vi "Intan_StreamData_64ch_parallelLoop.vi"(0 "VISA resource name":refnum<visa-resource-name>, 1 "refnum in":refnum<file>, 3 "stop":bool, 4 "Save Binary Data":bool, 5 "error in":errorcluster, 7 "byte order":T5(ring)=enum."little-endian", 8 "hdr fpath":path, 11 "DT_scale (sec)":dbl=0.01, 12 "aux file ref num":refnum<file>, 14 "save aux file":bool) -> (6 "N data scans to read (VISA)":i32=20, 10 "Nbytes VISA read":u32, 13 "VISA read iter":i32, 19 "error out":errorcluster)   [LabVIEW 2015]
doc: "Stream data to disk and user friendly display. Data is scaled and filtered prior to display.\n\nThis VI uses parallel while loop architecture: 1 loop reads from serial stream and saves raw bytes to disk; the other loop processes the data in chunk, scaling and filtering, then displays."
uses:
  zip_swcircularbuffer1_0_19b/Circular Buffer/Controls/Circular Buffer Status.ctl
  zip_swcircularbuffer1_0_19b/Circular Buffer/Controls/Circular Buffer Operations.ctl
  <vilib>/Utility/error.llb/DialogType.ctl
  zip_swcircularbuffer1_0_19b/Circular Buffer/Instance VIs/Circular Buffer(1D U16).vi
  zip_swcircularbuffer1_0_19b/Circular Buffer/Circular Buffer.lvlib
panel:
  out "A+B chans":i32[](array[numeric])
  out "Bchans":i32[](array[numeric])
  out "Achans":i32[](array[numeric])
  in  "Tab Control":T1(tab)
  in  "DisplayScale (uV/div)":u16(ring)=1 items=["6400", "3200", "1600", "800", "400", "200", "100", "50", "25"]
  in  "offset factor":dbl=1.0
  in  "Filter settings":T2={"LP Filter On/Off"=TRUE, "LP Cutoff (Hz)"=40.0, "HP Filter On/Off"=TRUE, "HP Cutoff (Hz)"=0.5, "Bandstop On/Off"=TRUE, "fl Cutoff (Hz)"=48.0, "fh Cutoff (Hz) "=52.0}
  out "Save status":bool
  out "non integer read":bool
  out "display iter":i32
  out "% buffer full":dbl(slide) scale=0.0..100.0
  in  "Ring Buffer Size":T3={"Samples per Channel"=640000, "Channels"=0}
  out "buffer underflow":bool
  out "Buffer Status  (read)":T4
  out "buffer overflow":bool
  out "Buffer Status (write)":T4
  in  "Center Traces":bool
  in  "Display Chans":i32[](listbox)=[1, 4, 13, 14, 15, 16, 17, 22]
  out "FS (Hz)":dbl
  in  "ChartDisplayLength (s)":dbl=5.0
  in  "Display Update interval (ms)":dbl=100.0
  in  "Buffer Read Interval (ms)":dbl=100.0
  in  "View Channels":u16(ring) items=["A and B (0-63)", "A chans (0-31)", "B chans (32-63)", "Free Select"]
  in  "bytes per scan":i32=140
  in  "Nchans":i32=64
  in  "start stream (Teensy char)":string="s"
  in  "pause stream (Teensy char)":string="p"
  out "Text response":string
  out "timestamp_array":i32[](array[numeric])
  out "aux_cmd_array":i32[][](array[numeric])
  out "binary data (from VISA read)":u16[](array[numeric])
  out "setscaleresult":dbl
  out "UpdateCode":i16
  out "xmax_init":dbl
  out "offset_init":dbl
  out "increment_init":dbl
  out "xmin_init":dbl
  out "NchansChanged":bool
  out "DispLengthChanged":bool
  out "XscaleRollover":bool
  out "error code out":i32 format="%0.0f"
  out "StopLoopsMaster":bool
  out "N_u16s  write to buf":i32
  out "Nelements to read from buf":dbl
  out "N data scans to display":u16=20
  out "YtxtLabelsAll":string[](array[string])
  out "Picture":picture
  out "Intan Streaming Data":dbl[][](graph)
  # "Intan-Teensy Bioelectric Module: Data Stream and Visualization"
  # "Display Settings"
  # "Ring Buffer Status"
  # "1-D data stream \nreformatted  to 2-D"
  # "xscale controls"
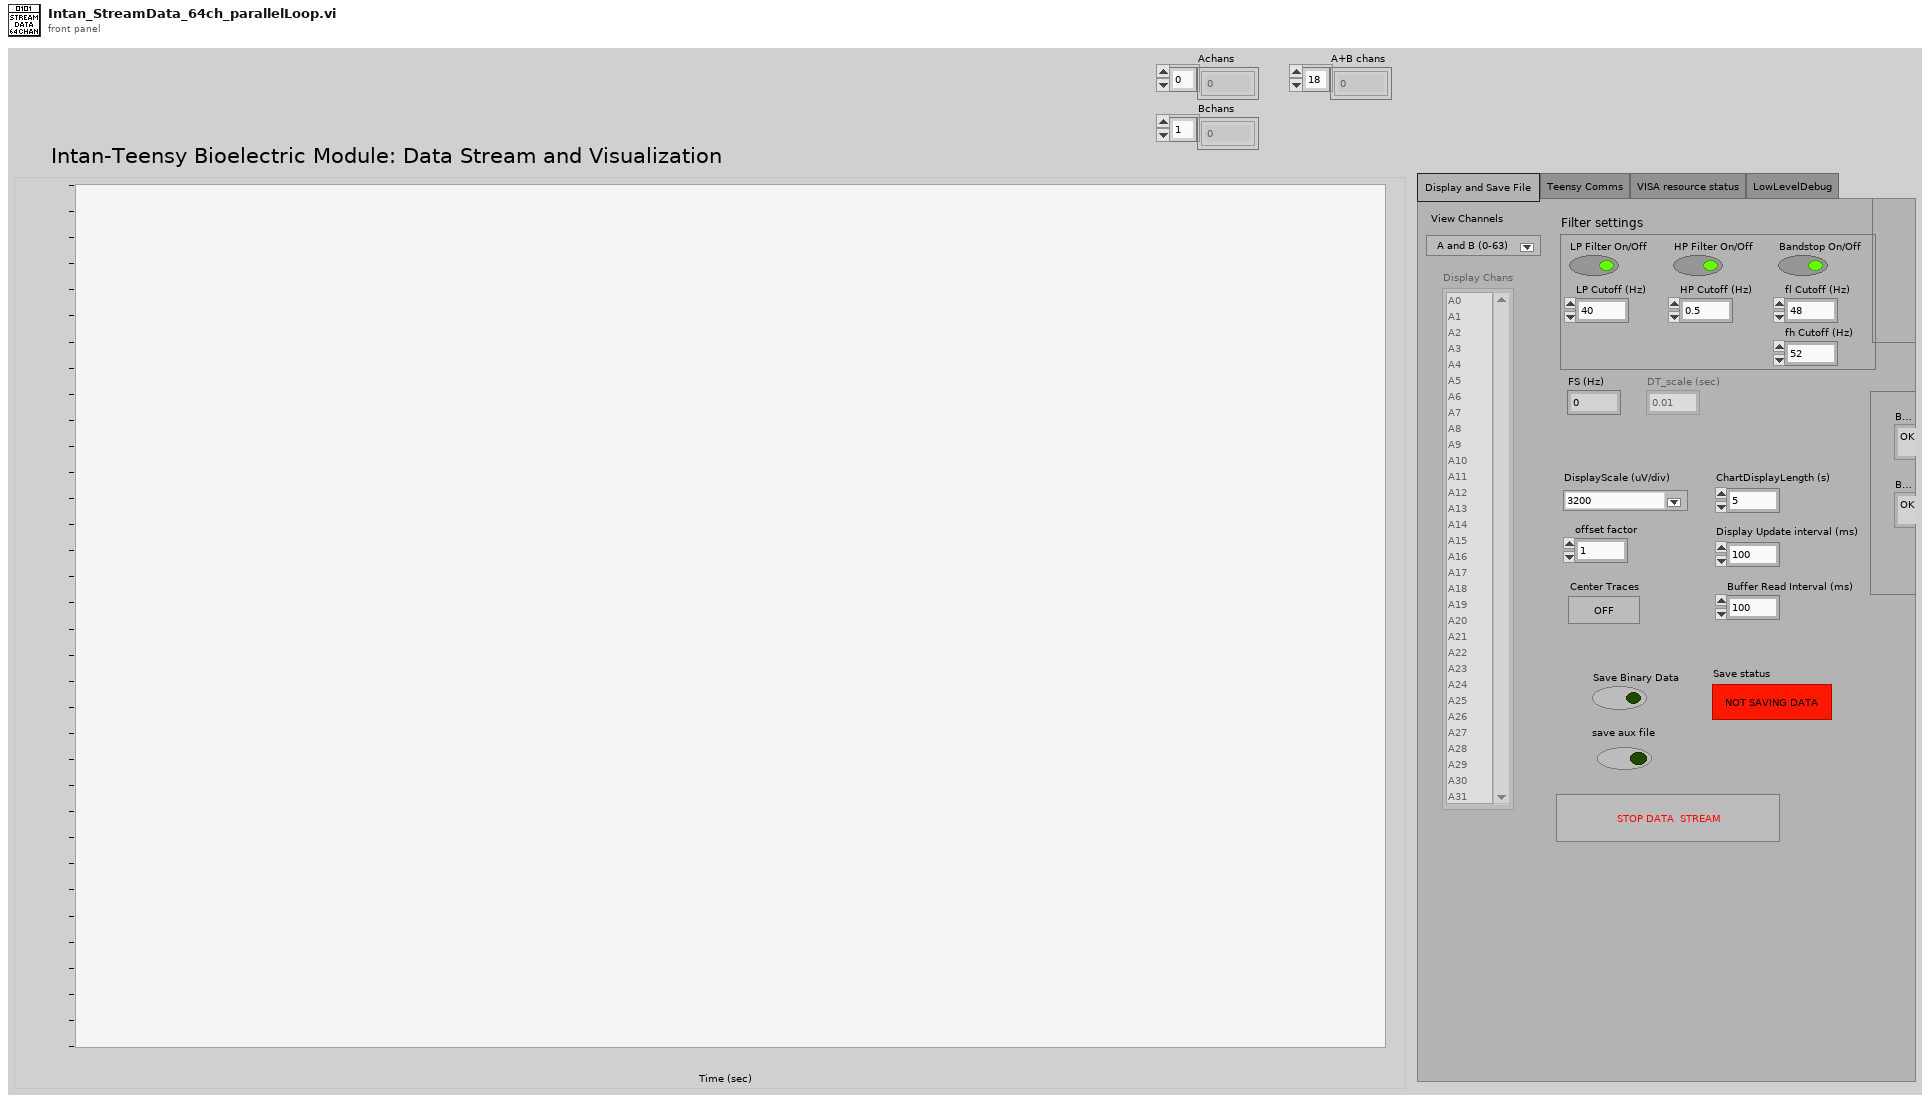
[diagram p1: front panel]
types:
  T1 = enum32{"Display and Save File ", "Teensy Comms", "VISA resource status", "LowLevelDebug"}
  T2 = cluster{"LP Filter On/Off":bool, "LP Cutoff (Hz)":dbl, "HP Filter On/Off":bool, "HP Cutoff (Hz)":dbl, "Bandstop On/Off":bool, "fl Cutoff (Hz)":dbl, "fh Cutoff (Hz) ":dbl}
  T3 = cluster{"Samples per Channel":u32, "Channels":u32}
  T4 = typedef "Circular Buffer.lvlib/Circular Buffer Status.ctl" = enum16{"OK", "Overflow", "Underflow"}
  T5 = enum16{"big-endian, network order", "native, host order", "little-endian"}
  T6 = typedef "Circular Buffer.lvlib/Circular Buffer Operations.ctl" = enum16{"Initialize", "Get Backlog", "Write", "Read (continuous)", "Read (most recent)"}
  T7 = enum8{"Enabled", "Disabled", "Disabled and Grayed Out"}
  T8 = typedef "LVRectTypeDef.ctl" = cluster{"Left":i16, "Top":i16, "Right":i16, "Bottom":i16}
  T9 = cluster{"XScale.Minimum":dbl, "XScale.Maximum":dbl, "XScale.Increment":dbl, "Nchannels":i32}
  T10 = cluster{"Maximum":dbl, dbl, dbl, dbl, dbl, dbl, "YscleMark":dbl, "Increment":dbl}
  T11 = typedef "DialogType.ctl" = u16
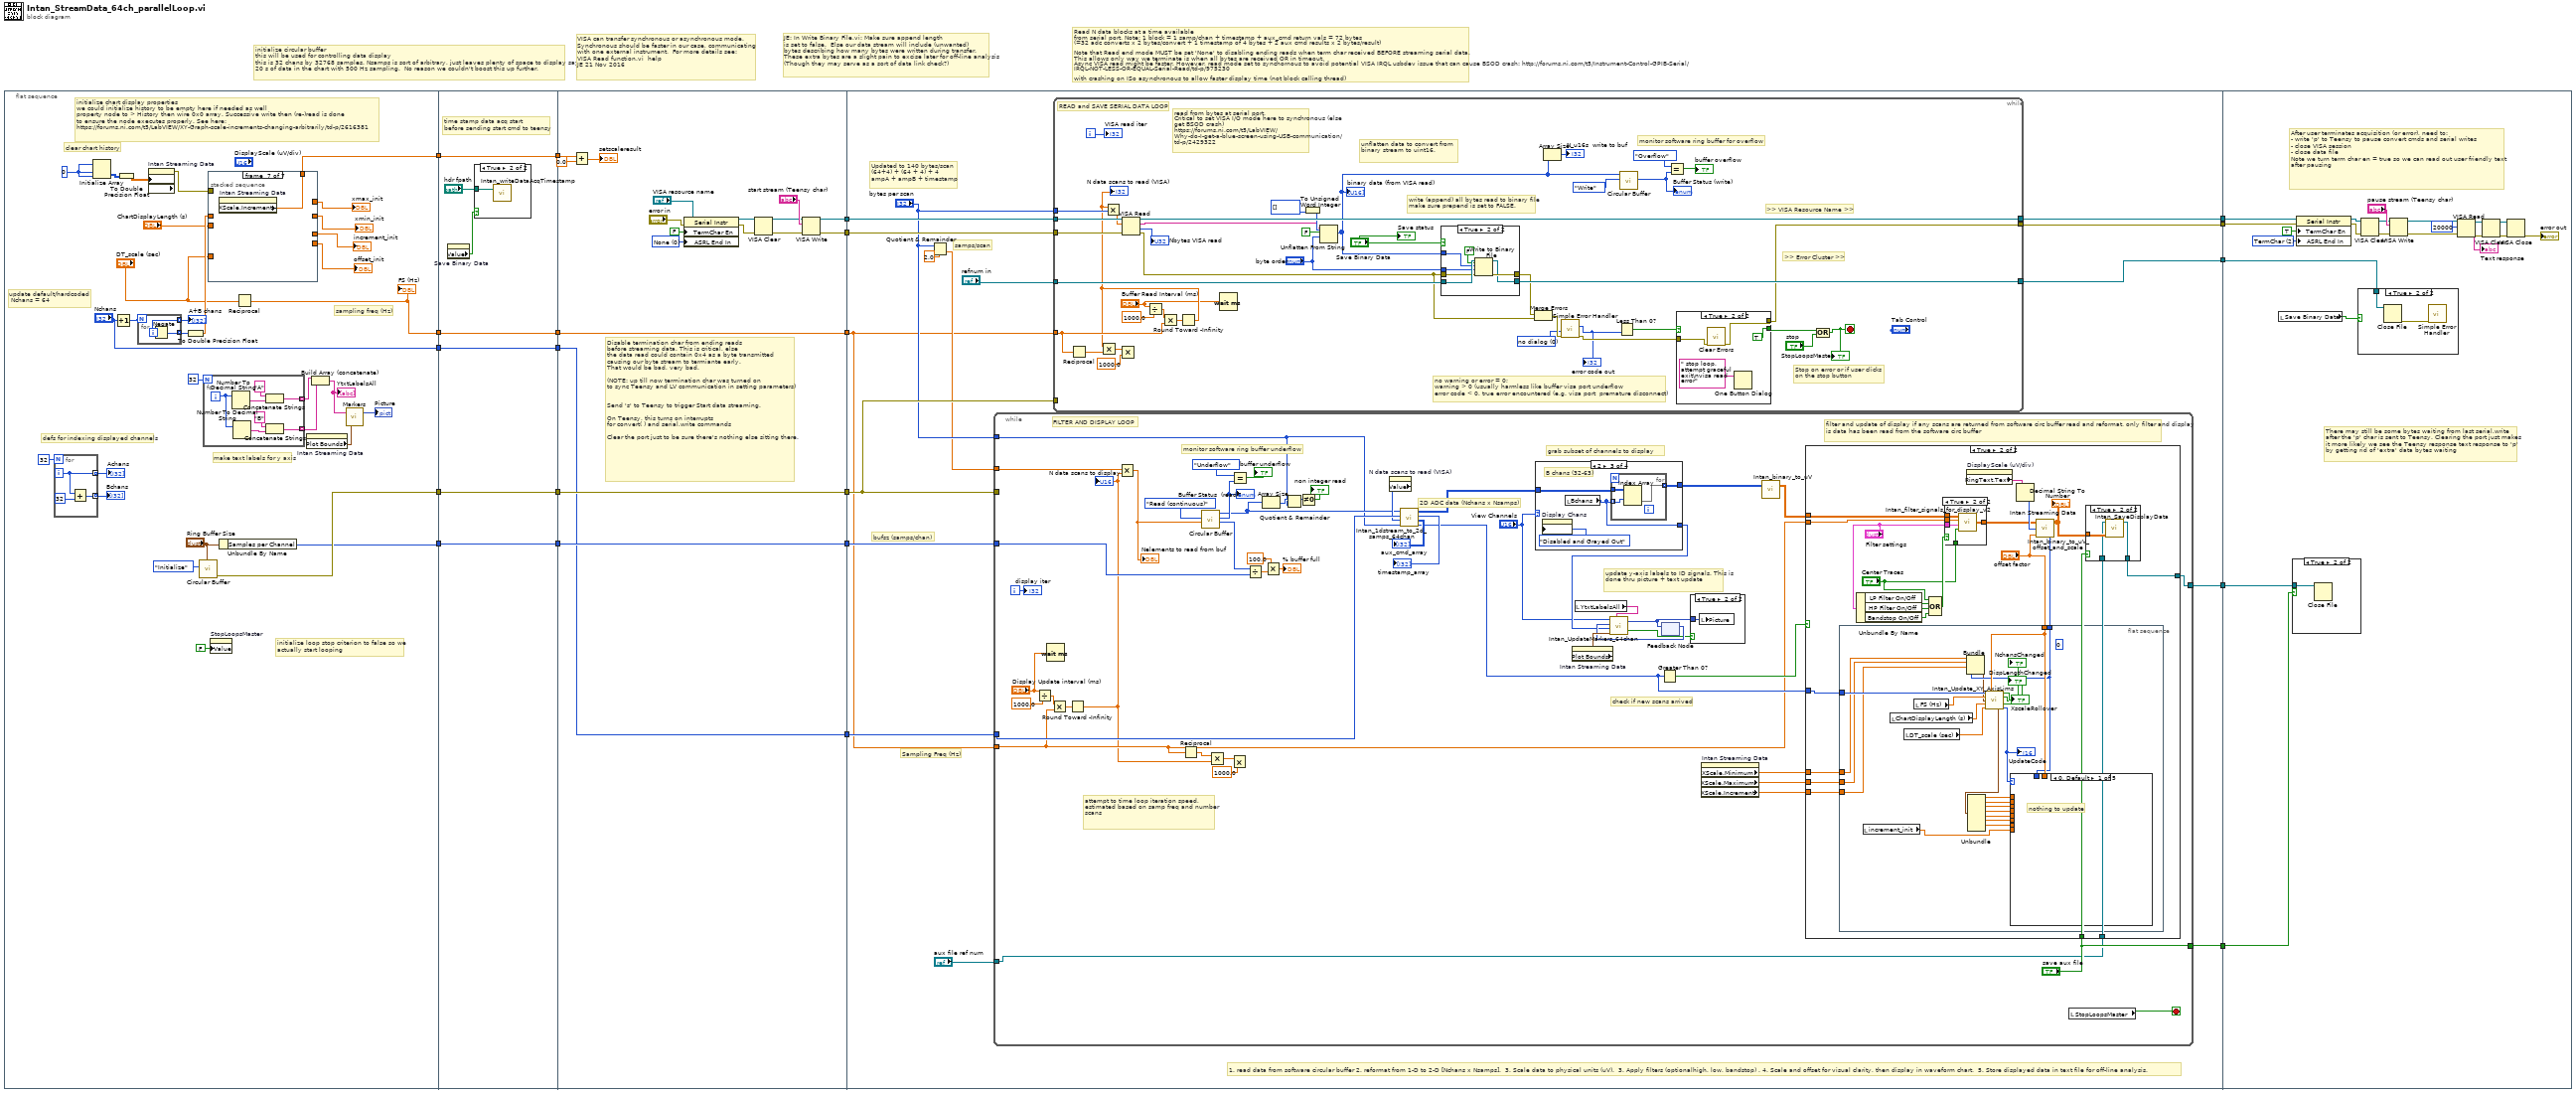
[diagram p0: block diagram]
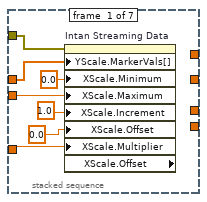
[diagram p2: hidden frame]
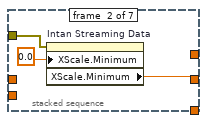
[diagram p3: hidden frame]
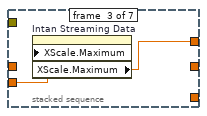
[diagram p4: hidden frame]
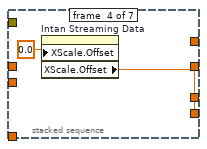
[diagram p5: hidden frame]
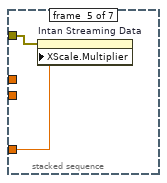
[diagram p6: hidden frame]
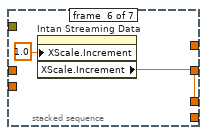
[diagram p7: hidden frame]
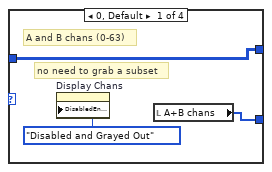
[diagram p10: hidden frame]
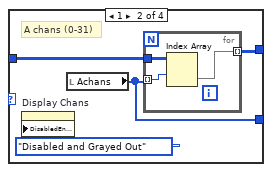
[diagram p11: hidden frame]
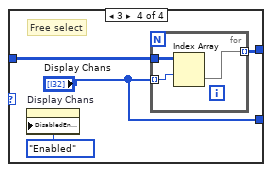
[diagram p12: hidden frame]
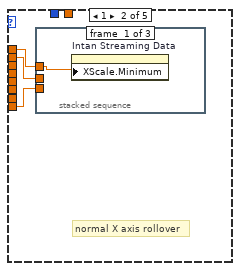
[diagram p14: hidden frame]
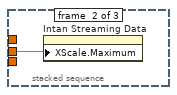
[diagram p15: hidden frame]
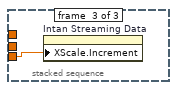
[diagram p16: hidden frame]
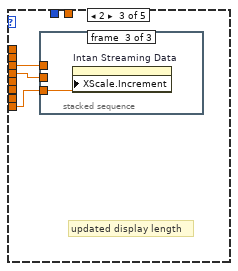
[diagram p17: hidden frame]
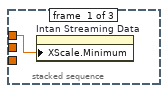
[diagram p18: hidden frame]
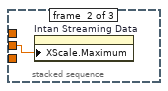
[diagram p19: hidden frame]
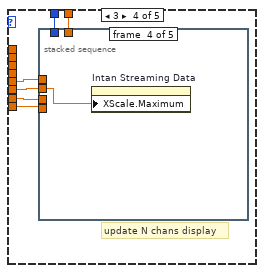
[diagram p20: hidden frame]
diagram:
  # "Read N data blocks at a time available\nfrom serial port. Note: 1 block = 1 samp/chan + timestamp + aux_cmd return vals = 72 bytes \n(=32 adc converts x 2 bytes/convert + 1 timestamp of 4 bytes + 2 aux cmd results x 2 bytes/result) \n\nNote that Read end mode MUST be set 'None' to disabling ending reads when term char received BEFORE streaming serial data.  \nThis allows only way we terminate is when all bytes are received OR in timeout.  \nAsync VISA read might be faster. However, read mode set to synchornous to avoid potential VISA IRQL usbdev issue that can cause BSOD crash: http://forums.ni.com/t5/Instrument-Control-GPIB-Serial/IRQL-NOT-LESS-OR-EQUAL-Serial-Read/td-p/975230\n\nwith crashing on ISo asynchronous to allow faster display time (not block calling thread)"
  # "initialize circular buffer\nthis will be used for controlling data display\nthis is 32 chans by 32768 samples. Nsamps is sort of arbitrary, just leaves plenty of space to display say\n20 s of data in the chart with 500 Hz sampling.  No reason we couldn't boost this up further."
  # "JE: In Write Binary File.vi: Make sure append length \nis set to false.  Else our data stream will include (unwanted)\nbytes describing how many bytes were written during transfer.\nThese extra bytes are a slight pain to excise later for off-line analysis\n(Though they may serve as a sort of data link check?)"
  # "VISA can transfer synchronous or asynchronous mode.\nSynchronous should be faster in our case, communicating\nwith one external instrument.  For more details see: \nVISA Read function.vi  help \nJE 21 Nov 2016"
  n1 = flat-sequence {
    tunnel: [w49] -> w10
    tunnel: [w47] -> w8
    tunnel: ["Nchans"] -> w6
    tunnel: [w42] -> w4
    tunnel: [w30] -> w2
    tunnel: w10 -> [w90]
    tunnel: [w90] -> w9
    tunnel: w8 -> [w89]
    tunnel: [w89] -> w7
    tunnel: w6 -> [w88]
    tunnel: [w88] -> w5
    tunnel: w4 -> [w87]
    tunnel: [w87] -> w3
    tunnel: w2 -> [w86]
    tunnel: [w86] -> w1
    tunnel: [w99] -> w19
    tunnel: [w100] -> w18
    tunnel: [w98] -> w17
    tunnel: w9 -> [w98]
    tunnel: [w97] -> w16
    tunnel: w7 -> [w97]
    tunnel: w5 -> [w96]
    tunnel: [w96] -> w15
    tunnel: [w95] -> w14
    tunnel: w3 -> [w95]
    tunnel: w1 -> [w94]
    tunnel: [w121] -> w21
    tunnel: [w124] -> w20
    tunnel: w19 -> [w122]
    tunnel: w18 -> [w123]
    tunnel: w17 -> [w120]
    tunnel: w16 -> [w118]
    tunnel: w15 -> [w117]
    tunnel: w14 -> [w114]
    tunnel: [w113] -> w13
    tunnel: [w111] -> w12
    tunnel: [w110] -> w11
    tunnel: w21 -> [w361]
    tunnel: w20 -> [w374]
    tunnel: w13 -> [w356]
    tunnel: w12 -> [w355]
    tunnel: w11 -> [w354]
    frame #0 {
      w41 = 0 ("Dimension Size")
      # "defs for indexing displayed channels"
      # "update default/hardcoded\n Nchans = 64"
      # "clear chart history"
      # "initialize loop stop criterion to false so we\nactually start looping"
      # "make text labels for y axis"
      # "sampling freq (Hz)"
      # "initialize chart display properties\nwe could initialize history to be empty here if needed as well\nproperty node to > History then wire 0x0 array. Successive write then (re-)read is done\nto ensure the node executes properly. See here:\nhttps://forums.ni.com/t5/LabVIEW/XY-Graph-scale-increments-changing-arbitrarily/td-p/2616381"
      n2 = for {
        N: 32 -> [_]
        tunnel: [w55] -> w28 mode=indexing
        tunnel: [w53] -> w27 mode=indexing
        i -> [w55]
        n3 = Add(x=w55, y=32) -> (x+y=w53:i32)
      }
      "Achans" <- w28
      "Bchans" <- w27
      n4 = Initialize Array(w41, w41, w41) -> (w40:i32[][])
      n5 = Increment(x="Nchans") -> (x+1=w51:i32)
      n6 = To Double Precision Float(number=w40) -> (double precision float=w38:dbl[][])
      n7 = for {
        N: w51 -> [_]
        tunnel: [w83] -> w52 mode=indexing
        tunnel: [w82] -> w26 mode=indexing
        i -> [w82]
        n8 = Negate(x=w82) -> (-x=w83:i32)
      }
      "A+B chans" <- w26
      n9 = property on="Intan Streaming Data" class="WFChart (strict)" props=["History Data", "History Data"]("History Data"=w38) -> (error out=w37:errorcluster)  [unwired: 2 in, 2 out]
      n10 = To Double Precision Float(number=w52) -> (double precision float=w39:dbl[])
      n11 = call-poly "Circular Buffer.vi"("Buffer Size"="Ring Buffer Size", "Operation"=Circular_Buffer_Operations."Initialize") -> ("error out"=w49:errorcluster)  [unwired: 6 in, 3 out]
      n12 = for {
        N: 32 -> [_]
        tunnel: [w79] -> w24 mode=indexing
        tunnel: [w75] -> w23 mode=indexing
        i -> [w76]
        n13 = Number To Decimal String(number=w76) -> (decimal integer string=w81:string)  [unwired: 1 in]
        n14 = Number To Decimal String(number=w76) -> (decimal integer string=w78:string)  [unwired: 1 in]
        n15 = Concatenate Strings("A" ("string"), w81) -> (w79:string)
        n16 = Concatenate Strings("B" ("string"), w78) -> (w75:string)
      }
      n17 = stacked-sequence {
        tunnel: w39 -> [w62 _ _ _ _ _ _]
        tunnel: w37 -> [w61 w64 _ _ w70 _ _]
        tunnel: "ChartDisplayLength (s)" -> [w59 _ w67 _ _ _ _]
        tunnel: "DT_scale (sec)" -> [w58 _ _ _ w71 _ _]
        tunnel: [_ _ w66 _ _ _ _] -> w31
        tunnel: [_ w65 _ _ _ _ _] -> w34
        tunnel: [_ _ _ _ _ w72 _] -> w33
        tunnel: [_ _ _ w68 _ _ _] -> w32
        tunnel: [_ _ _ _ _ _ w74] -> w30
        frame #0 {
          n18 = property on="Intan Streaming Data" class="WFChart (strict)" props=["YScale", "MarkerVals[]", "XScale", "Minimum", "XScale", "Maximum", "XScale", "Increment", "XScale", "Offset", "XScale", "Multiplier", "XScale", "Offset"](error in=w61, "YScale.MarkerVals[]"=w62, "XScale.Minimum"=0.0 ("X Scale.Range:Minimum"), "XScale.Maximum"=w59, "XScale.Increment"=1.0 ("X Scale.Range:Minimum"), "XScale.Offset"=0.0 ("X Scale.Range:Minimum"), "XScale.Multiplier"=w58) -> ()  [unwired: 1 in, 3 out]
        }
        frame #1 {
          n19 = property on="Intan Streaming Data" class="WFChart (strict)"(error in=w64, "XScale.Minimum"=0.0 ("X Scale.Range:Minimum")) -> ("XScale.Minimum"=w65:dbl)  [unwired: 1 in, 2 out]
        }
        frame #2 {
          n20 = property on="Intan Streaming Data" class="WFChart (strict)"("XScale.Maximum"=w67) -> ("XScale.Maximum"=w66:dbl)  [unwired: 2 in, 2 out]
        }
        frame #3 {
          n21 = property on="Intan Streaming Data" class="WFChart (strict)"("XScale.Offset"=0.0 ("X Scale.Offset and Multiplier:Offset")) -> ("XScale.Offset"=w68:dbl)  [unwired: 2 in, 2 out]
        }
        frame #4 {
          n22 = property on="Intan Streaming Data" class="WFChart (strict)"(error in=w70, "XScale.Multiplier"=w71) -> ()  [unwired: 1 in, 2 out]
        }
        frame #5 {
          n23 = property on="Intan Streaming Data" class="WFChart (strict)"("XScale.Increment"=1.0 ("X Scale.Range:Increment")) -> ("XScale.Increment"=w72:dbl)  [unwired: 2 in, 2 out]
        }
        frame #6 {
          n24 = property on="Intan Streaming Data" class="WFChart (strict)"() -> ("XScale.Increment"=w74:dbl)  [unwired: 2 in, 2 out]
        }
      }
      "xmin_init" <- w34
      "increment_init" <- w33
      "offset_init" <- w32
      "xmax_init" <- w31
      n25 = property on="StopLoopsMaster" class="Bool (strict)"("Value"=FALSE ("StopLoopsMaster")) -> ()  [unwired: 2 in, 2 out]
      n26 = Unbundle By Name("Ring Buffer Size") -> ("Samples per Channel"=w47:u32)
      n27 = Reciprocal(x="DT_scale (sec)") -> (1/x=w42:dbl)
      "FS (Hz)" <- w42
      n28 = property on="Intan Streaming Data" class="WFChart (strict)"() -> ("Plot Bounds"=w43:T8)  [unwired: 2 in, 2 out]
      n29 = Build Array (concatenate)(w24, w23) -> (w22:string[])
      "YtxtLabelsAll" <- w22
      n30 = call "Markers.vi"("plot bounds"=w43, "Array"=w22) -> ("Picture"=→"Picture":picture)  [unwired: 1 out]
    }
    frame #1 {
      # "time stamp data acq start\nbefore sending start cmd to teensy"
      n31 = property on="Save Binary Data" class="Bool (strict)"() -> ("Value"=w85:bool)  [unwired: 2 in, 2 out]
      n32 = case shown="True" w85 {
        tunnel: "hdr fpath" -> [_ w91]
        frame False {
        }
        frame True {
          n33 = call "Intan_writeDataAcqTimestamp.vi"("hdr fpath"=w91) -> ()  [unwired: 2 in, 1 out]
        }
      }
    }
    frame #2 {
      w105 = u16 0 items=["None", "Last Bit", "TermChar"] ("Serial Settings:End Mode for Reads")
      # "Disable termination char from ending reads\nbefore streaming data. This is critical, else\nthe data read could contain 0x4 as a byte transmitted\ncausing our byte stream to termiante early.\nThat would be bad, very bad.\n\n(NOTE: up till now termination char was turned on\nto sync Teensy and LV communication in setting parameters)\n\n\nSend 's' to Teensy to trigger Start data streaming.  \n\nOn Teensy, this turns on interrupts\nfor convert( ) and serial.write commands\n\nClear the port just to be sure there's nothing else sitting there."
      n34 = Add(x=w94, y=0.0) -> (x+y=→"setscaleresult":dbl)
      n35 = property class="Serial Instr"(reference="VISA resource name", error in="error in", "TermChar En"=FALSE ("Message Based Settings:Termination Character Enable"), "ASRL End In"=w105) -> (reference out=w104:refnum<visa-resource-name>, error out=w103:errorcluster)
      n36 = VISA Clear(VISA resource name=w104, error in (no error)=w103) -> (VISA resource name out=w102:refnum<visa-resource-name>, error out=w101:errorcluster)
      n37 = VISA Write(VISA resource name=w102, write buffer="start stream (Teensy char)", error in (no error)=w101) -> (VISA resource name out=w100:refnum<visa-resource-name>, error out=w99:errorcluster)  [unwired: 1 out]
    }
    frame #3 {
      # "Updated to 140 bytes/scan\n(64+4) + (64 + 4) + 4\nampA + ampB + timestamp"
      # "1. read data from software circular buffer 2. reformat from 1-D to 2-D [Nchans x Nsamps].  3. Scale data to physical units (uV).  3. Apply filters (optionalhigh, low, bandstop) . 4. Scale and offset for visual clarity, then display in waveform chart.  5. Store displayed data in text file for off-line analysis."
      # "Sampling Freq (Hz)"
      # "bufsz (samps/chan)"
      # "samps/scan"
      n38 = Quotient & Remainder(x="bytes per scan", y=2.0) -> (floor(x/y)=w115:dbl)  [unwired: 1 out]
      n39 = while {
        tunnel: w120 -> [_]
        tunnel: w118 -> [w169]
        tunnel: w117 -> [w165]
        tunnel: "bytes per scan" -> [w155]
        tunnel: w114 -> [w136]
        tunnel: w115 -> [w161]
        tunnel: [w142] -> w113
        tunnel: "aux file ref num" -> [w141]
        tunnel: ["save aux file"] -> w110
        i -> [w162]
        stop <- w139 stop-if-true
        # "2D ADC data (Nchans x Nsamps)"
        # "check if new scans arrived"
        # "grab subset of channels to display"
        # "update y-axis labels to ID signals. This is done thru picture + text update"
        # "FILTER AND DISPLAY LOOP"
        # "attempt to time loop iteration speed,\nestimated based on samp freq and number scans"
        # "filter and update of display if any scans are returned from software circ buffer read and reformat. only filter and display is data has been read from the software circ buffer"
        # "monitor software ring buffer underflow"
        n40 = Divide(x="Display Update interval (ms)", y=1000.0) -> (x/y=w133:dbl)
        n41 = Wait (ms)(milliseconds to wait="Display Update interval (ms)") -> ()  [unwired: 1 out]
        n42 = Multiply(x=w133, y=w136) -> (x*y=w135:dbl)
        n43 = Round Toward -Infinity(1:w135) -> (0:w134:dbl)
        "N data scans to display" <- w134
        n44 = Multiply(x=w161, y=w134) -> (x*y=w160:dbl)
        "Nelements to read from buf" <- w160
        n45 = Reciprocal(x=w136) -> (1/x=w152:dbl)
        n46 = call-poly "Circular Buffer.vi"("Read Size"=w160, "Operation"=Circular_Buffer_Operations."Read (continuous)") -> ("Elements Remaining"=w170:i32, "Buffer Status"=w172:T4, "Data Out"=w157:u16[])  [unwired: 6 in, 1 out]
        "Buffer Status  (read)" <- w172
        n47 = Multiply(x=w152, y=w134) -> (x*y=w151:dbl)
        n48 = Multiply(x=w151, y=1000.0) -> ()  [unwired: 1 out]
        n49 = Equal?(x=Circular_Buffer_Status."Underflow" ("y"), y=w172) -> (x = y?=→"buffer underflow":bool)
        n50 = Divide(x=w170, y=w169) -> (x/y=w168:dbl)
        n51 = Array Size(array=w157) -> (size(s)=w156:i32)
        n52 = Multiply(x=100.0, y=w168) -> (x*y=→"% buffer full":dbl)
        n53 = Quotient & Remainder(x=w156, y=w155) -> (x-y*floor(x/y)=w154:i32)  [unwired: 1 out]
        n54 = Not Equal To 0?(x=w154) -> (x != 0?=→"non integer read":bool)
        n55 = property on="N data scans to read (VISA)" class="DigNum (strict)"() -> ("Value"=w159:i32)  [unwired: 2 in, 2 out]
        n56 = call "Intan_1dstream_to_2d_samps_64chan.vi"("bytes per scan"=w155, "N data scans to read"=w159, "Nchans"=w165, "1-D  data in"=w157) -> ("Nscans read"=w140:i32, "aux_cmd_array A_and_B"=→"aux_cmd_array":i16[][], "timestamp_array"=→"timestamp_array":i32[], "2d ADCdata_array out_ampA_and_B"=w149:u16[][])  [unwired: 2 in, 2 out]
        n57 = case shown="2" "View Channels" {
          tunnel: w149 -> [w178 w182 w189 w196]
          tunnel: [w178 w181 w188 w195] -> w138
          tunnel: [w176 w179 w186 "Display Chans"] -> w127
          frame 0, Default {
            # "A and B chans (0-63)"
            # "no need to grab a subset"
            n58 = property on="Display Chans" class="LstBox (strict)"("DisabledEnum"=T7."Disabled and Grayed Out" ("Disabled")) -> ()  [unwired: 2 in, 2 out]
            n59 = local read "A+B chans"() -> (w176:i32[])
          }
          frame 1 {
            # "A chans (0-31)"
            n60 = property on="Display Chans" class="LstBox (strict)"("DisabledEnum"=T7."Disabled and Grayed Out" ("Disabled")) -> ()  [unwired: 2 in, 2 out]
            n61 = local read "Achans"() -> (w179:i32[])
            n62 = for {
              tunnel: w182 -> [w185]
              tunnel: w179 -> [w183] mode=indexing
              tunnel: [w184] -> w181 mode=indexing
              n63 = Index Array(array=w185, index (row)=w183) -> (element=w184:u16[])  [unwired: 1 in]
            }
          }
          frame 2 {
            # "B chans (32-63)"
            n64 = property on="Display Chans" class="LstBox (strict)"("DisabledEnum"=T7."Disabled and Grayed Out" ("Disabled")) -> ()  [unwired: 2 in, 2 out]
            n65 = local read "Bchans"() -> (w186:i32[])
            n66 = for {
              tunnel: w189 -> [w192]
              tunnel: w186 -> [w190] mode=indexing
              tunnel: [w191] -> w188 mode=indexing
              n67 = Index Array(array=w192, index (row)=w190) -> (element=w191:u16[])  [unwired: 1 in]
            }
          }
          frame 3 {
            # "Free select"
            n68 = property on="Display Chans" class="LstBox (strict)"("DisabledEnum"=T7."Enabled" ("Disabled")) -> ()  [unwired: 2 in, 2 out]
            n69 = for {
              tunnel: w196 -> [w199]
              tunnel: "Display Chans" -> [w197] mode=indexing
              tunnel: [w198] -> w195 mode=indexing
              n70 = Index Array(array=w199, index (row)=w197) -> (element=w198:u16[])  [unwired: 1 in]
            }
          }
        }
        n71 = property on="Intan Streaming Data" class="WFChart (strict)"() -> ("Plot Bounds"=w147:T8)  [unwired: 2 in, 2 out]
        n72 = local read "YtxtLabelsAll"() -> (w137:string[])
        n73 = Greater Than 0?(x=w140) -> (x > 0?=w158:bool)
        n74 = feedback #1() -> (w146:picture)  [unwired: 1 in]
        n75 = call "Intan_UpdateMarkers_64chan.vi"("ChanSelectMode"="View Channels", "Picture In"=w146, "Display Chans"=w127, "plot bounds"=w147, "YtxtLabelsAll"=w137) -> ("Picture Out"=w144:picture, "update labels"=w145:bool)
        n76 = feedback-in #1(w144) -> ()
        n77 = case shown="True" w145 {
          tunnel: w144 -> [_ w175]
          frame False {
          }
          frame True {
            n78 = local write "Picture"(w175) -> ()
          }
        }
        n79 = property on="Intan Streaming Data" class="WFChart (strict)"() -> ("XScale.Minimum"=w130:dbl, "XScale.Maximum"=w129:dbl, "XScale.Increment"=w128:dbl)  [unwired: 2 in, 2 out]
        n80 = call "Intan_binary_to_uV.vi"("2d ADC binary data"=w138) -> ("Scaled Data (uV)"=w148:dbl[][])  [unwired: 2 in]
        n81 = case shown="True" w158 {
          tunnel: w136 -> [_ w220]
          tunnel: w148 -> [_ w218]
          tunnel: [w200 w211] -> w142
          tunnel: "save aux file" -> [_ w210]
          tunnel: w141 -> [w200 w209]
          tunnel: w140 -> [_ w207]
          tunnel: w130 -> [_ w203]
          tunnel: w129 -> [_ w202]
          tunnel: w128 -> [_ w201]
          frame False {
          }
          frame True {
            n82 = flat-sequence {
              tunnel: w207 -> [w242]
              tunnel: "offset factor" -> [w229]
              tunnel: w204 -> [w226]
              tunnel: w203 -> [w224]
              tunnel: w202 -> [w223]
              tunnel: w201 -> [w222]
              frame #0 {
                (unwired) 0 ("index")
                n83 = local read "increment_init"() -> (w228:dbl)
                n84 = local read "ChartDisplayLength (s)"() -> (w240:dbl)
                n85 = local read "DT_scale (sec)"() -> (w239:dbl)
                n86 = local read "FS (Hz)"() -> (w241:dbl)
                n87 = Bundle("XScale.Minimum"=w224, "XScale.Maximum"=w223, "XScale.Increment"=w222, "Nchannels"=w226) -> (w225:T9)  [unwired: 1 in]
                n88 = call "Intan_Update_XY_AxisLims.vi"("NscansRead"=w242, "offset factor"=w229, "FS (Hz)"=w241, "XscaleClusterCurrent"=w225, "DisplayLength(s)"=w240, "DT_scale (s)"=w239) -> ("XscaleRollover"=→"XscaleRollover":bool, "DispLengthChanged"=→"DispLengthChanged":bool, "NchansChanged"=→"NchansChanged":bool, "XYlims Update Cluster"=w237:T10, "UpdateCode"=w238:i16)  [unwired: 4 in, 1 out]
                "UpdateCode" <- w238
                n89 = Unbundle(w237) -> ("Maximum"=w234:dbl, w233:dbl, w231:dbl, w230:dbl, w236:dbl, w235:dbl, "YscleMark"=w232:dbl)  [unwired: 1 out]
                n90 = case shown="0, Default" w238 {
                  tunnel: w226 -> [_ _ _ w262 w273]
                  tunnel: w236 -> [_ _ _ w257 _]
                  tunnel: w235 -> [_ _ _ w261 _]
                  tunnel: w234 -> [_ w247 _ _ w276]
                  tunnel: w233 -> [_ w246 _ _ w275]
                  tunnel: w232 -> [_ _ _ w260 w274]
                  tunnel: w231 -> [_ _ w252 _ _]
                  tunnel: w230 -> [_ _ w253 _ _]
                  tunnel: w229 -> [_ _ _ w259 w272]
                  tunnel: w228 -> [_ w245 w251 w258 w271]
                  frame 0, Default {
                    # "nothing to update"
                  }
                  frame 1 {
                    # "normal X axis rollover"
                    n91 = stacked-sequence {
                      tunnel: w247 -> [w248 _ _]
                      tunnel: w246 -> [_ w249 _]
                      tunnel: w245 -> [_ _ w250]
                      frame #0 {
                        n92 = property on="Intan Streaming Data" class="WFChart (strict)"("XScale.Minimum"=w248) -> ()  [unwired: 2 in, 2 out]
                      }
                      frame #1 {
                        n93 = property on="Intan Streaming Data" class="WFChart (strict)"("XScale.Maximum"=w249) -> ()  [unwired: 2 in, 2 out]
                      }
                      frame #2 {
                        n94 = property on="Intan Streaming Data" class="WFChart (strict)"("XScale.Increment"=w250) -> ()  [unwired: 2 in, 2 out]
                      }
                    }
                  }
                  frame 2 {
                    # "updated display length"
                    n95 = stacked-sequence {
                      tunnel: w251 -> [_ _ w256]
                      tunnel: w253 -> [_ w255 _]
                      tunnel: w252 -> [w254 _ _]
                      frame #0 {
                        n96 = property on="Intan Streaming Data" class="WFChart (strict)"("XScale.Minimum"=w254) -> ()  [unwired: 2 in, 2 out]
                      }
                      frame #1 {
                        n97 = property on="Intan Streaming Data" class="WFChart (strict)"("XScale.Maximum"=w255) -> ()  [unwired: 2 in, 2 out]
                      }
                      frame #2 {
                        n98 = property on="Intan Streaming Data" class="WFChart (strict)"("XScale.Increment"=w256) -> ()  [unwired: 2 in, 2 out]
                      }
                    }
                  }
                  frame 3 {
                    # "update N chans display"
                    n99 = stacked-sequence {
                      tunnel: w262 -> [w266 _ _ _ _]
                      tunnel: w258 -> [_ _ _ _ w270]
                      tunnel: w261 -> [_ _ _ w269 _]
                      tunnel: w260 -> [_ _ _ _ _]
                      tunnel: w259 -> [w264 _ _ _ _]
                      tunnel: w257 -> [_ w267 w268 _ _]
                      frame #0 {
                        n100 = Negate(x=w266) -> (-x=w265:i32)
                        n101 = Multiply(x=w264, y=w265) -> (x*y=w263:dbl)
                        n102 = property on="Intan Streaming Data" class="WFChart (strict)"("YScale.Minimum"=w263) -> ()  [unwired: 2 in, 2 out]
                      }
                      frame #1 {
                        n103 = property on="Intan Streaming Data" class="WFChart (strict)"("XScale.Offset"=w267) -> ()  [unwired: 2 in, 2 out]
                      }
                      frame #2 {
                        n104 = property on="Intan Streaming Data" class="WFChart (strict)"("XScale.Minimum"=w268) -> ()  [unwired: 2 in, 2 out]
                      }
                      frame #3 {
                        n105 = property on="Intan Streaming Data" class="WFChart (strict)"("XScale.Maximum"=w269) -> ()  [unwired: 2 in, 2 out]
                      }
                      frame #4 {
                        n106 = property on="Intan Streaming Data" class="WFChart (strict)"("XScale.Increment"=w270) -> ()  [unwired: 2 in, 2 out]
                      }
                    }
                  }
                  frame 4 {
                    # "updated offset factor"
                    n107 = stacked-sequence {
                      seq-local: [w277 _ _] -> [_ w281 _]
                      tunnel: w276 -> [_ _ _]
                      tunnel: w275 -> [_ _ _]
                      tunnel: w274 -> [_ _ _]
                      tunnel: w273 -> [w280 _ _]
                      tunnel: w272 -> [w278 _ _]
                      tunnel: w271 -> [_ _ w286]
                      frame #0 {
                        n108 = Negate(x=w280) -> (-x=w279:i32)
                        n109 = Multiply(x=w278, y=w279) -> (x*y=w277:dbl)
                        n110 = property on="Intan Streaming Data" class="WFChart (strict)"("YScale.Minimum"=w277) -> ()  [unwired: 2 in, 2 out]
                      }
                      frame #1 {
                        n111 = for {
                          N: w281 -> [_]
                          tunnel: [w284] -> w283 mode=indexing
                          i -> [w285]
                          n112 = Negate(x=w285) -> (-x=w284:i32)
                        }
                        n113 = To Double Precision Float(number=w283) -> (double precision float=w282:dbl[])
                        n114 = property on="Intan Streaming Data" class="WFChart (strict)" props=["YScale", "MarkerVals[]", "YScale", "MarkerVals[]"]("YScale.MarkerVals[]"=w282) -> ()  [unwired: 2 in, 3 out]
                      }
                      frame #2 {
                        n115 = property on="Intan Streaming Data" class="WFChart (strict)"("XScale.Increment"=w286) -> ()  [unwired: 2 in, 2 out]
                      }
                    }
                  }
                }
              }
            }
            n116 = Unbundle By Name("Filter settings") -> ("LP Filter On/Off"=w216:bool, "HP Filter On/Off"=w215:bool, "Bandstop On/Off"=w213:bool)
            n117 = Compound Arithmetic op=OR("Center Traces", w216, w215, w213) -> (w214:bool)
            n118 = case shown="True" w214 {
              tunnel: w220 -> [_ w296]
              tunnel: w218 -> [w291 w295]
              tunnel: [w291 w294] -> w208
              tunnel: "Filter settings" -> [_ w293]
              tunnel: "Center Traces" -> [_ w292]
              frame False {
              }
              frame True {
                n119 = call "Intan_filter_signals_for_display_v2.vi"("Center Traces"=w292, "input filter cluster"=w293, "Sample Rate (Hz)"=w296, "Nchan Array In [Nchans x Nsamps]"=w295) -> ("Display Signals Out [Nchans x Nsamps]"=w294:dbl[][])
              }
            }
            n120 = property on="DisplayScale (uV/div)" class="Ring (strict)"() -> ("RingText.Text"=w219:string)  [unwired: 2 in, 2 out]
            n121 = Decimal String To Number(string=w219) -> (number=w221:i32)  [unwired: 2 in, 1 out]
            n122 = call "Intan_binary_to_uV_offset_and_scale.vi"("offset spacing factor"="offset factor", "Yscale (uv/div)"=w221, "ScaledData [Nchans x Nsamps]"=w208) -> ("Nchannels"=w204:i32, "Data4Display"=w206:dbl[][])  [unwired: 1 in]
            "Intan Streaming Data" <- w206
            n123 = case shown="True" w210 {
              tunnel: w206 -> [_ w290]
              tunnel: [w287 w289] -> w211
              tunnel: w209 -> [w287 w288]
              frame False {
              }
              frame True {
                n124 = call "Intan_SaveDisplayData.vi"("2d ADCdata_array out"=w290, "aux file ref num"=w288) -> ("refnum out"=w289:refnum<file>)  [unwired: 3 in]
              }
            }
          }
        }
        n125 = local read "StopLoopsMaster"() -> (w139:bool)
        "display iter" <- w162
      }
      n126 = while {
        tunnel: [w337] -> w121
        tunnel: [w335] -> w124
        tunnel: w122 -> [w331]
        tunnel: "refnum in" -> [w334]
        tunnel: w123 -> [w332]
        tunnel: w120 -> [_]
        tunnel: "bytes per scan" -> [w316]
        tunnel: w114 -> [w299]
        tunnel: [w303] -> w111
        i -> [w333]
        stop <- w336 stop-if-true
        w309 = T11 0 items=["no dialog", "OK message", "continue or stop message", "OK message + warnings", "continue/stop + warnings"] ("type of dialog (OK msg:1)")
        # "no warning or error = 0;\nwarning > 0 (usually harmless like buffer visa port underflow\nerror code < 0, true error encountered (e.g. visa port  premature disconnect)"
        # "READ and SAVE SERIAL DATA LOOP"
        # "monitor software ring buffer for overflow"
        # "write (append) all bytes read to binary file\nmake sure prepend is set to FALSE."
        # "unflatten data to convert from binary stream to uint16."
        # "Stop on error or if user clicks \non the stop button"
        # ">> Error Cluster >>"
        # ">> VISA Resource Name >>"
        # "read from bytes at serial port.\nCritical to set VISA I/O mode here to synchronous (else get BSOD crash)\nhttps://forums.ni.com/t5/LabVIEW/Why-do-I-get-a-blue-screen-using-USB-communication/td-p/2429322"
        n127 = Reciprocal(x=w299) -> (1/x=w313:dbl)
        n128 = Divide(x="Buffer Read Interval (ms)", y=1000.0) -> (x/y=w301:dbl)
        n129 = Multiply(x=w301, y=w299) -> (x*y=w302:dbl)
        n130 = Round Toward -Infinity(1:w302) -> (0:w298:dbl)
        "N data scans to read (VISA)" <- w298
        n131 = Multiply(x=w298, y=w313) -> (x*y=w315:dbl)
        n132 = Multiply(x=w298, y=w316) -> (x*y=w317:dbl)
        n133 = Multiply(x=w315, y=1000.0) -> ()  [unwired: 1 out]
        n134 = VISA Read(VISA resource name=w332, byte count=w317, error in (no error)=w331) -> (VISA resource name out=w337:refnum<visa-resource-name>, read buffer=w325:string, return count=→"Nbytes VISA read":u32, error out=w311:errorcluster)
        n135 = Wait (ms)(milliseconds to wait="Buffer Read Interval (ms)") -> ()  [unwired: 1 out]
        n136 = To Unsigned Word Integer(number=i16[] []) -> (unsigned 16bit integer=w327:u16[])
        n137 = Unflatten From String(type=w327, binary string=w325, data includes array or string size? (T)=FALSE, byte order (0:big-endian, network order)="byte order") -> (value=w319:u16[])  [unwired: 1 in, 2 out]
        "binary data (from VISA read)" <- w319
        n138 = case shown="True" "Save Binary Data" {
          tunnel: [w345 w352] -> w312
          tunnel: [w344 w351] -> w335
          tunnel: w334 -> [w344 w350]
          tunnel: w311 -> [w345 w349]
          tunnel: "byte order" -> [_ w347]
          tunnel: w319 -> [_ w346]
          frame False {
          }
          frame True {
            n139 = Write to Binary File(file (use dialog)=w350, data=w346, error in=w349, 5:FALSE ("prepend array or string size? (T)"), 9:w347) -> (refnum out=w351:refnum<file>, error out=w352:errorcluster)  [unwired: 1 in, 1 out]
          }
        }
        n140 = Merge Errors(w312, w311) -> (w310:errorcluster)
        n141 = Array Size(array=w319) -> (size(s)=→"N_u16s  write to buf":i32)
        n142 = call <vilib>:"Simple Error Handler.vi"("type of dialog (OK msg:1)"=w309, "error in (no error)"=w310) -> ("code out"=w306:i32, "error out"=w307:errorcluster)  [unwired: 3 in, 3 out]
        "error code out" <- w306
        n143 = Less Than 0?(x=w306) -> (x < 0?=w304:bool)
        n144 = call-poly "Circular Buffer.vi"("Operation"=Circular_Buffer_Operations."Write", "Data In"=w319) -> ("Buffer Status"=w321:T4)  [unwired: 6 in, 3 out]
        "Buffer Status (write)" <- w321
        n145 = Equal?(x=Circular_Buffer_Status."Overflow" ("y"), y=w321) -> (x = y?=→"buffer overflow":bool)
        n146 = case shown="True" w304 {
          tunnel: w307 -> [w338 w342]
          tunnel: [FALSE TRUE] -> w305
          tunnel: [w338 w340] -> w303
          frame False {
          }
          frame True {
            n147 = call <vilib>:"Clear Errors.vi"("error in (no error)"=w342) -> ("error out"=w340:errorcluster)  [unwired: 5 in, 1 out]
            n148 = One Button Dialog(message=" stop loop, attempt graceful exit\nvisa read error") -> ()  [unwired: 1 in, 1 out]
          }
        }
        n149 = Compound Arithmetic op=OR(w305, "stop") -> (w336:bool)
        "StopLoopsMaster" <- w336
        "VISA read iter" <- w333
        "Save status" <- "Save Binary Data"
      }
    }
    frame #4 {
      w366 = u16 2 items=["None", "Last Bit", "TermChar"] ("Serial Settings:End Mode for Reads")
      # "There may still be some bytes waiting from last serial.write\nafter the 'p' char is sent to Teensy. Clearing the port just makes\nit more likely we see the Teensy response text response to 'p' \nby getting rid of 'extra' data bytes waiting"
      # "After user terminates acquisition (or error), need to:\n- write 'p' to Teensy to pause convert cmds and serial writes\n- close VISA session\n- close data file\nNote we turn term char en = true so we can read out user friendly text \nafter pausing"
      n150 = local read "Save Binary Data"() -> (w353:bool)
      n151 = case shown="True" w354 {
        tunnel: w356 -> [_ w377]
        frame False {
        }
        frame True {
          n152 = Close File(refnum=w377) -> ()  [unwired: 1 in, 2 out]
        }
      }
      n153 = property class="Serial Instr"(reference=w361, error in=w355, "TermChar En"=TRUE ("Message Based Settings:Termination Character Enable"), "ASRL End In"=w366) -> (reference out=w360:refnum<visa-resource-name>, error out=w359:errorcluster)
      n154 = case shown="True" w353 {
        tunnel: w374 -> [_ w375]
        frame False {
        }
        frame True {
          n155 = Close File(refnum=w375) -> (error out=w376:errorcluster)  [unwired: 1 in, 1 out]
          n156 = call <vilib>:"Simple Error Handler.vi"("error in (no error)"=w376) -> ()  [unwired: 4 in, 5 out]
        }
      }
      n157 = VISA Clear(VISA resource name=w360, error in (no error)=w359) -> (VISA resource name out=w358:refnum<visa-resource-name>, error out=w357:errorcluster)
      n158 = VISA Write(VISA resource name=w358, write buffer="pause stream (Teensy char)", error in (no error)=w357) -> (VISA resource name out=w369:refnum<visa-resource-name>, error out=w368:errorcluster)  [unwired: 1 out]
      n159 = VISA Read(VISA resource name=w369, byte count=u32 20000, error in (no error)=w368) -> (VISA resource name out=w365:refnum<visa-resource-name>, read buffer=→"Text response":string, error out=w363:errorcluster)  [unwired: 1 out]
      n160 = VISA Clear(VISA resource name=w365, error in (no error)=w363) -> (VISA resource name out=w364:refnum<visa-resource-name>, error out=w362:errorcluster)
      n161 = VISA Close(VISA resource name=w364, error in (no error)=w362) -> (error out=→"error out":errorcluster)
    }
  }
